vi "MGI Search Text for Tokens.vi"(2 "Token[i]":string[](array[string]), 3 "Text":string) -> (0 "Found i":i32, 1 "Match Found":bool)   [LabVIEW 2020]
doc: "Search the specified string starting at the specified offset for the one of the specified matches. The behavior enum effects the seaerch as follows:\n<B>Earliest Pattern</B>: Iterate all specified match patterns and use the one that occurs closest to the specified offset is used. \n<B>Prioritized Pattern</B>: Use the first match pattern in the array that is found anywhere in the string.\n<B>Earliest Replica</B>\n<B>Prioritized Replica</B>\nThe index of the match pattern is output\n\nAuthored by Shawn Walpole\nsupport@mooregoodideas.com\nwww.mooregoodideas.com\n\nCopyright (c) 2010, Moore Good Ideas, Inc.\n\nAll rights reserved.\n\nRedistribution and use in source and binary forms, with or without modification, are permitted provided that the following conditions are met:\n\n * Redistributions of source code must retain the above copyright notice, this list of conditions and the following disclaimer.\n * Redistributions in binary form must reproduce the above copyright notice, this list of conditions and the following disclaimer in the documentation and/or other materials provided with the distribution.\n * Neither the name of Moore Good Ideas, Inc. nor the names of its contributors may be used to endorse or promote products derived from this software without specific prior written permission.\n\nTHIS SOFTWARE IS PROVIDED BY THE COPYRIGHT HOLDERS AND CONTRIBUTORS \"AS IS\" AND ANY EXPRESS OR IMPLIED WARRANTIES, INCLUDING, BUT NOT LIMITED TO, THE IMPLIED WARRANTIES OF MERCHANTABILITY AND FITNESS FOR A PARTICULAR PURPOSE ARE DISCLAIMED. IN NO EVENT SHALL THE COPYRIGHT OWNER OR CONTRIBUTORS BE LIABLE FOR ANY DIRECT, INDIRECT, INCIDENTAL, SPECIAL, EXEMPLARY, OR CONSEQUENTIAL DAMAGES (INCLUDING, BUT NOT LIMITED TO, PROCUREMENT OF SUBSTITUTE GOODS OR SERVICES; LOSS OF USE, DATA, OR PROFITS; OR BUSINESS INTERRUPTION) HOWEVER CAUSED AND ON ANY THEORY OF LIABILITY, WHETHER IN CONTRACT, STRICT LIABILITY, OR TORT (INCLUDING NEGLIGENCE OR OTHERWISE) ARISING IN ANY WAY OUT OF THE USE OF THIS SOFTWARE, EVEN IF ADVISED OF THE POSSIBILITY OF SUCH DAMAGE.\n\nFreeware from Moore Good Ideas, www.mooregoodideas.com. Do not remove this line."
panel:
  in  "Token Match":enum16{"Pattern", "Exact"}(ring)
  in  "Search Type":enum16{"1st in Text", "1st in Token[]"}(ring)
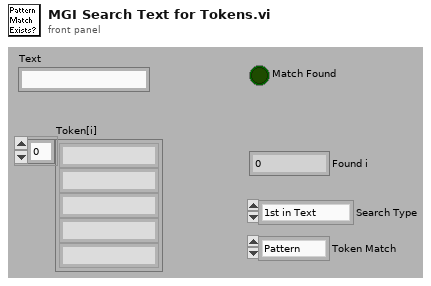
[diagram p1: front panel]
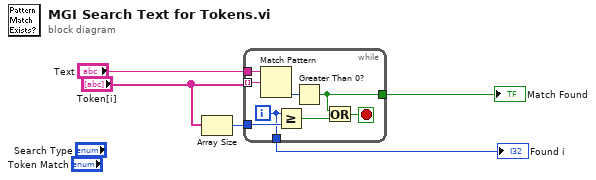
[diagram p0: block diagram]
diagram:
  n1 = Array Size(array="Token[i]") -> (size(s)=w3:i32)
  n2 = while {
    tunnel: "Text" -> [w13]
    tunnel: "Token[i]" -> [w12] mode=indexing
    tunnel: [w9] -> w4
    tunnel: w3 -> [w8]
    tunnel: [w6] -> w5
    i -> [w6]
    stop <- w10 stop-if-true
    n3 = Match Pattern(string=w13, regular expression=w12) -> (offset past match=w11:i32)  [unwired: 4 out]
    n4 = Greater Or Equal?(x=w6, y=w8) -> (x >= y?=w7:bool)
    n5 = Greater Than 0?(x=w11) -> (x > 0?=w9:bool)
    n6 = Or(x=w9, y=w7) -> (x .or. y?=w10:bool)
  }
  "Found i" <- w5
  "Match Found" <- w4
